vi "Write WebSocket Data Msg.vi"(10 "WebSocket Actor.lvlib:WebSocket Data Msg.lvclass":refnum<class "WebSocket Data Handler Msg.lvclass">, 11 "WebSocket Connection in":refnum<class "WebSocket Connection.lvclass">) -> (3 "WebSocket Connection out":refnum<class "WebSocket Connection.lvclass">)   [LabVIEW 2016, in "WebSocket Actor.lvlib" / "WebSocket Connection.lvclass"]
uses:
  WebSocket Connection.lvclass
  Abstract Messages/WebSocket Data Handler Msg/WebSocket Data Handler Msg.lvclass
  WebSocket Connection.lvclass/WebSocket Connection.ctl
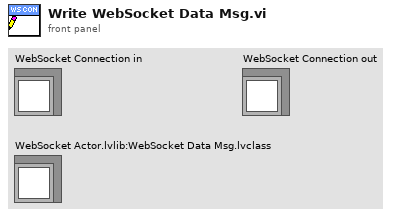
[diagram p1: front panel]
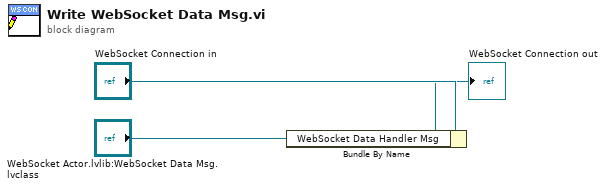
[diagram p0: block diagram]
diagram:
  n1 = Bundle By Name(cluster="WebSocket Connection in", "WebSocket Data Handler Msg"="WebSocket Actor.lvlib:WebSocket Data Msg.lvclass") -> (→"WebSocket Connection out":refnum<class "WebSocket Connection.lvclass">)
